vi "Connect.vi"(8 "error in (no error)":errorcluster, 10 "Channel(s)":string, 11 "SWITCH in":refnum<class "SWITCH.lvclass">) -> (0 "error out":errorcluster, 3 "SWITCH out":refnum<class "SWITCH.lvclass">)   [LabVIEW 2024, in "HAL_Example.lvlib" / "SWITCH.lvclass"]
uses:
  SWITCH.lvclass
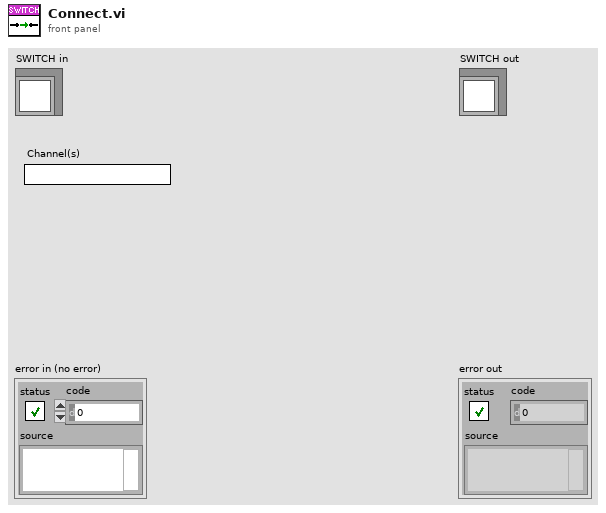
[diagram p1: front panel]
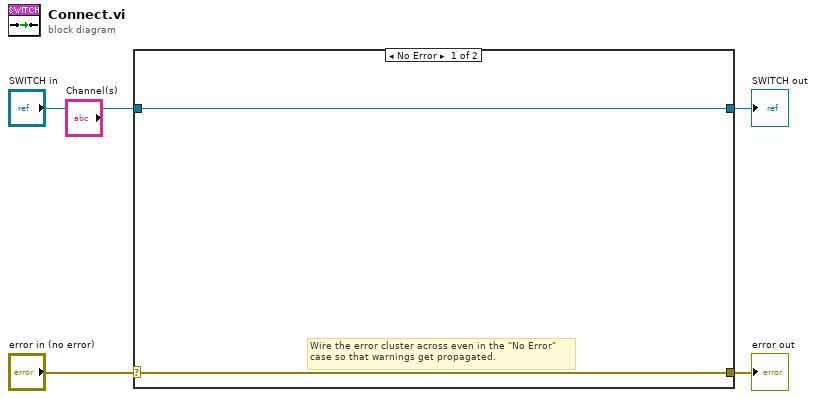
[diagram p0: block diagram]
diagram:
  n1 = case shown="No Error" "error in (no error)" {
    selector: "error in (no error)" -> [w5 w8]
    tunnel: [w5 w8] -> w3
    tunnel: [w6 w7] -> w1
    tunnel: "SWITCH in" -> [w6 w7]
    frame No Error {
      # "Wire the error cluster across even in the \"No Error\"\ncase so that warnings get propagated."
    }
    frame Error {
    }
  }
  "error out" <- w3
  "SWITCH out" <- w1
